vi "SendUpstreamMessage.vi"(8 "error in (no error)":errorcluster, 10 "UpstreamMsg":refnum<class "UpstreamMsgParent.lvclass">, 11 "ServiceManager-Comms in":refnum<class "ServiceManager-Comms.lvclass">) -> (0 "error out":errorcluster, 3 "ServiceManager-Comms out":refnum<class "ServiceManager-Comms.lvclass">)   [LabVIEW 2020, in "ServiceManager-Comms.lvlib" / "ServiceManager-Comms.lvclass"]
uses:
  ServiceManager-Comms.lvclass
  UpstreamMsg/UpstreamMsgParent/UpstreamMsgParent.lvclass
  ServiceManager-Comms.lvclass/ServiceManager-Comms.ctl
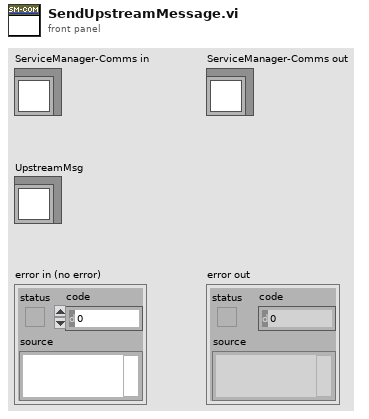
[diagram p1: front panel]
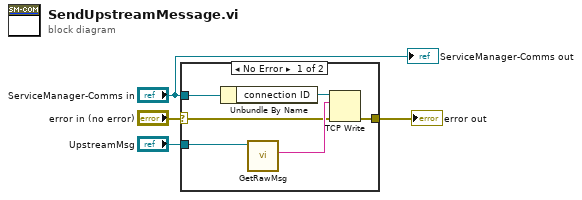
[diagram p0: block diagram]
diagram:
  n1 = case shown="No Error" "error in (no error)" {
    selector: "error in (no error)" -> [w6 w11]
    tunnel: "UpstreamMsg" -> [w10 _]
    tunnel: "ServiceManager-Comms in" -> [w9 _]
    tunnel: [w5 w11] -> w1
    frame No Error {
      n2 = Unbundle By Name(w9) -> ("connection ID"=w8:refnum<k5>)
      n3 = call-dynamic "GetRawMsg.vi"("UpstreamMsgParent in"=w10) -> ("Msg"=w7:string)  [unwired: 8 in, 2 out]
      n4 = TCP Write(connection ID=w8, data in=w7, error in (no error)=w6) -> (error out=w5:errorcluster)  [unwired: 1 in, 2 out]
    }
    frame Error {
    }
  }
  "error out" <- w1
  "ServiceManager-Comms out" <- "ServiceManager-Comms in"
